vi "Test.vi"(10 "Test Controls":T1 {"Belts" scale=-1.0..1.0; "Arm" scale=-1.0..1.0; "Drive Train" scale=-1.0..1.0}, 11 "Call Context":T9) -> (0 "Loop 2 Data":T5, 1 "SubState 2":T4, 2 "Loop 1 Data":T6, 3 "SubState 1":T4, 4 "SubState 3":T4, 5 "Loop 0 Data":T7, 6 "Loop 3 Data":T3, 7 "SubState 0":T4=enum."driver control", 8 "SubState 4":T8, 9 "Test Data":T2)   [LabVIEW 2013]
uses:
  typedefs/subStates.ctl
  <vilib>/Rock Robotics/WPI/DriverStation/WPI_DriverStationDerivedRobotMode.ctl
  typedefs/singleUseSubstate.ctl
  typedefs/Loop Datatypes/Loop 0 Datatype.ctl
  typedefs/Loop Datatypes/Loop 1 Datatype.ctl
  typedefs/Loop Datatypes/Loop 2 Datatype.ctl
  typedefs/Loop Datatypes/Loop 3 Datatype.ctl
  typedefs/test/test data.ctl
  typedefs/test/test controls.ctl
  typedefs/fg_typedef.ctl
  typedefs/DevRef Type.ctl
  <vilib>/Rock Robotics/WPI/Solenoid/WPI_SolenoidGetEnum.vi
  <vilib>/Rock Robotics/WPI/Joystick/WPI_JoystickGetSetRefNum.vi
panel:
  out "JS Axis-X":dbl
  out "JS Axis-Y":dbl
  out "Exit Value":i32=-1
  # "Loop Data and Substates"
  # "Drive Loop"
  # "State Machine Master Loop"
  # "Pickup/Passing Belts Loop"
  # "Pickup/Passing Arm Loop"
  # "Pneumatics Loop"
  # "Test Code (Only Run in Test Mode)"
  # "Pneumatics"
  # "Home Encoders"
  # "Manual Override"
  # "Joystick Control"
  # "Arm Safeties"
  # "Sensors"
  # "Drive Encoders"
  # "Pneumatics Commands"
  # "Arm Encoder"
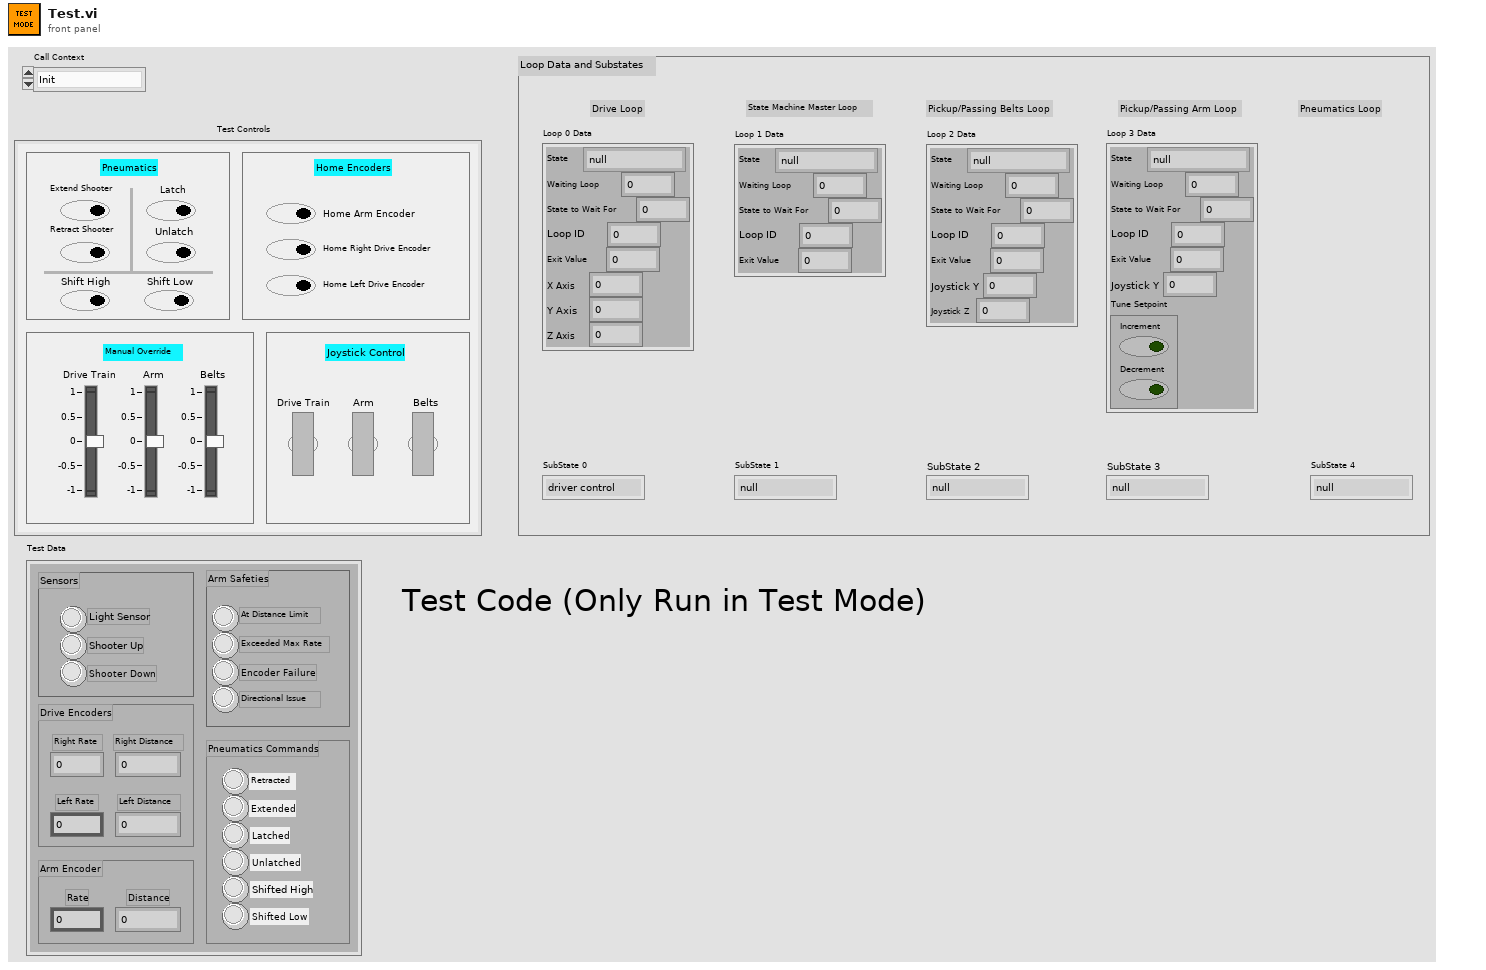
[diagram p1: front panel]
types:
  T1 = typedef "test controls.ctl" = cluster{"Drive Train":dbl, "Arm":dbl, "Belts":dbl, "Drive Train":bool, "Arm":bool, "Belts":bool, "Home Arm Encoder":bool, "Home Right Drive Encoder":bool, "Home Left Drive Encoder":bool, "Extend Shooter":bool, "Retract Shooter":bool, "Latch":bool, "Unlatch":bool, "Shift High":bool, "Shift Low":bool}
  T2 = typedef "test data.ctl" = cluster{"Light Sensor":bool, "Shooter Up":bool, "Shooter Down":bool, "Left Rate":dbl, "Left Distance":dbl, "Right Rate":dbl, "Right Distance":dbl, "Rate":dbl, "Distance":dbl, "At Distance Limit":bool, "Exceeded Max Rate":bool, "Encoder Failure":bool, "Directional Issue":bool, "Latched":bool, "Unlatched":bool, "Shifted High":bool, "Shifted Low":bool, "Extended":bool, "Retracted":bool}
  T3 = typedef "Loop 3 Datatype.ctl" = cluster{"State":T4, "Waiting Loop":i32, "State to Wait For":i32, "Loop ID":i32, "Exit Value":i32, "Joystick Y":dbl, "Tune Setpoint":cluster{"Increment":bool, "Decrement":bool}}
  T4 = typedef "subStates.ctl" = enum16{"null", "wait", "driver control", "auto", "manual override", "hold position", "rotate", "pickup", "pass", "load", "goto shoot", "shoot high goal", "shoot low goal", "cancel arm", "cancel shooter", "end", "test"}
  T5 = typedef "Loop 2 Datatype.ctl" = cluster{"State":T4, "Waiting Loop":i32, "State to Wait For":i32, "Loop ID":i32, "Exit Value":i32, "Joystick Y":dbl, "Joystick Z":dbl}
  T6 = typedef "Loop 1 Datatype.ctl" = cluster{"State":T4, "Waiting Loop":i32, "State to Wait For":i32, "Loop ID":i32, "Exit Value":i32}
  T7 = typedef "Loop 0 Datatype.ctl" = cluster{"State":T4, "Waiting Loop":i32, "State to Wait For":i32, "Loop ID":i32, "Exit Value":i32, "X Axis":dbl, "Y Axis":dbl, "Z Axis":dbl}
  T8 = typedef "singleUseSubstate.ctl" = enum16{"null", "wait", "shift high", "shift low", "extend shooter", "retract shooter", "latch", "unlatch", "end"}
  T9 = typedef "WPI_DriverStationDerivedRobotMode.ctl" = enum16{"Init", "Execute", "Stop"}
  T10 = typedef "DevRef Type.ctl" = enum16{"Shooter Solenoid", "Latch Solenoid", "Right Up Sensor", "Right Down Sensor", "Hold Sensor", "2 Ball Switch", "Arm Encoder"}
  T11 = typedef "fg_typedef.ctl" = enum16{"Get", "Set"}
  T12 = typedef "WPI_EncoderDevRef.ctl" = cluster{"DevStatus":errorcluster, "EncoderIndex":T13, "CounterIndex":T14, "DistancePerCount":dbl, "Decoding Type":T15}
  T13 = typedef "FPGA_EncoderIdx.ctl" = enum8{"Enc 0", "Enc 1", "Enc 2", "Enc 3", "Invalid"}
  T14 = typedef "FPGA_CounterCtrSystemIndex.ctl" = enum8{"Ctr 0", "Ctr 1", "Ctr 2", "Ctr 3", "Ctr 4", "Ctr 5", "Ctr 6", "Ctr 7", "Invalid"}
  T15 = typedef "WPI_EncoderType.ctl" = enum16{"1x", "2x", "4x"}
  T16 = typedef "dashboard safety status data.ctl" = cluster{"At Distance Limit":bool, "Encoder Error":bool, "Excedded Rate Limit":bool, "Encoder Directional Issue":bool}
  T17 = typedef "WPI_SolenoidDevRef.ctl" = cluster{"DevStatus":errorcluster, "Solenoid Module":T18, "Forward Solenoid Channel":T19, "Reverse Solenoid Channel":T19}
  T18 = typedef "FPGA_TypedefSolenoidModule.ctl" = enum16{"Solenoid Module 1", "Solenoid Module 2"}
  T19 = typedef "WPI_SolenoidChannel.ctl" = enum8{"Solenoid 1", "Solenoid 2", "Solenoid 3", "Solenoid 4", "Solenoid 5", "Solenoid 6", "Solenoid 7", "Solenoid 8", "Invalid"}
  T20 = typedef "WPI_DigitalInputDevRef.ctl" = cluster{"DevStatus":errorcluster, "DIO Channel":T21, "Digital Module":T22}
  T21 = typedef "FPGA_DIOChannel.ctl" = enum8{"DIO 1", "DIO 2", "DIO 3", "DIO 4", "DIO 5", "DIO 6", "DIO 7", "DIO 8", "DIO 9", "DIO 10", "DIO 11", "DIO 12", "DIO 13", "DIO 14", "Invalid"}
  T22 = typedef "FPGA_TypedefDigitalModule.ctl" = enum16{"Digital Module 1", "Digital Module 2"}
  T23 = typedef "WPI_JoystickDevRef.ctl" = cluster{"Device":T24}
  T24 = typedef "WPI_JoystickDeviceEnum.ctl" = enum16{"USB 1", "USB 2", "USB 3", "USB 4", "Kinect 1", "Kinect 2"}
  T25 = cluster{"axis 1 (x)":dbl, "axis 2 (y)":dbl, "axis 3 (throttle)":dbl, "axis 4":dbl, "axis 5":dbl, "axis 6":dbl}
  T26 = typedef "WPI_SolenoidValue.ctl" = enum16{"Off", "On", "Forward", "Reverse"}
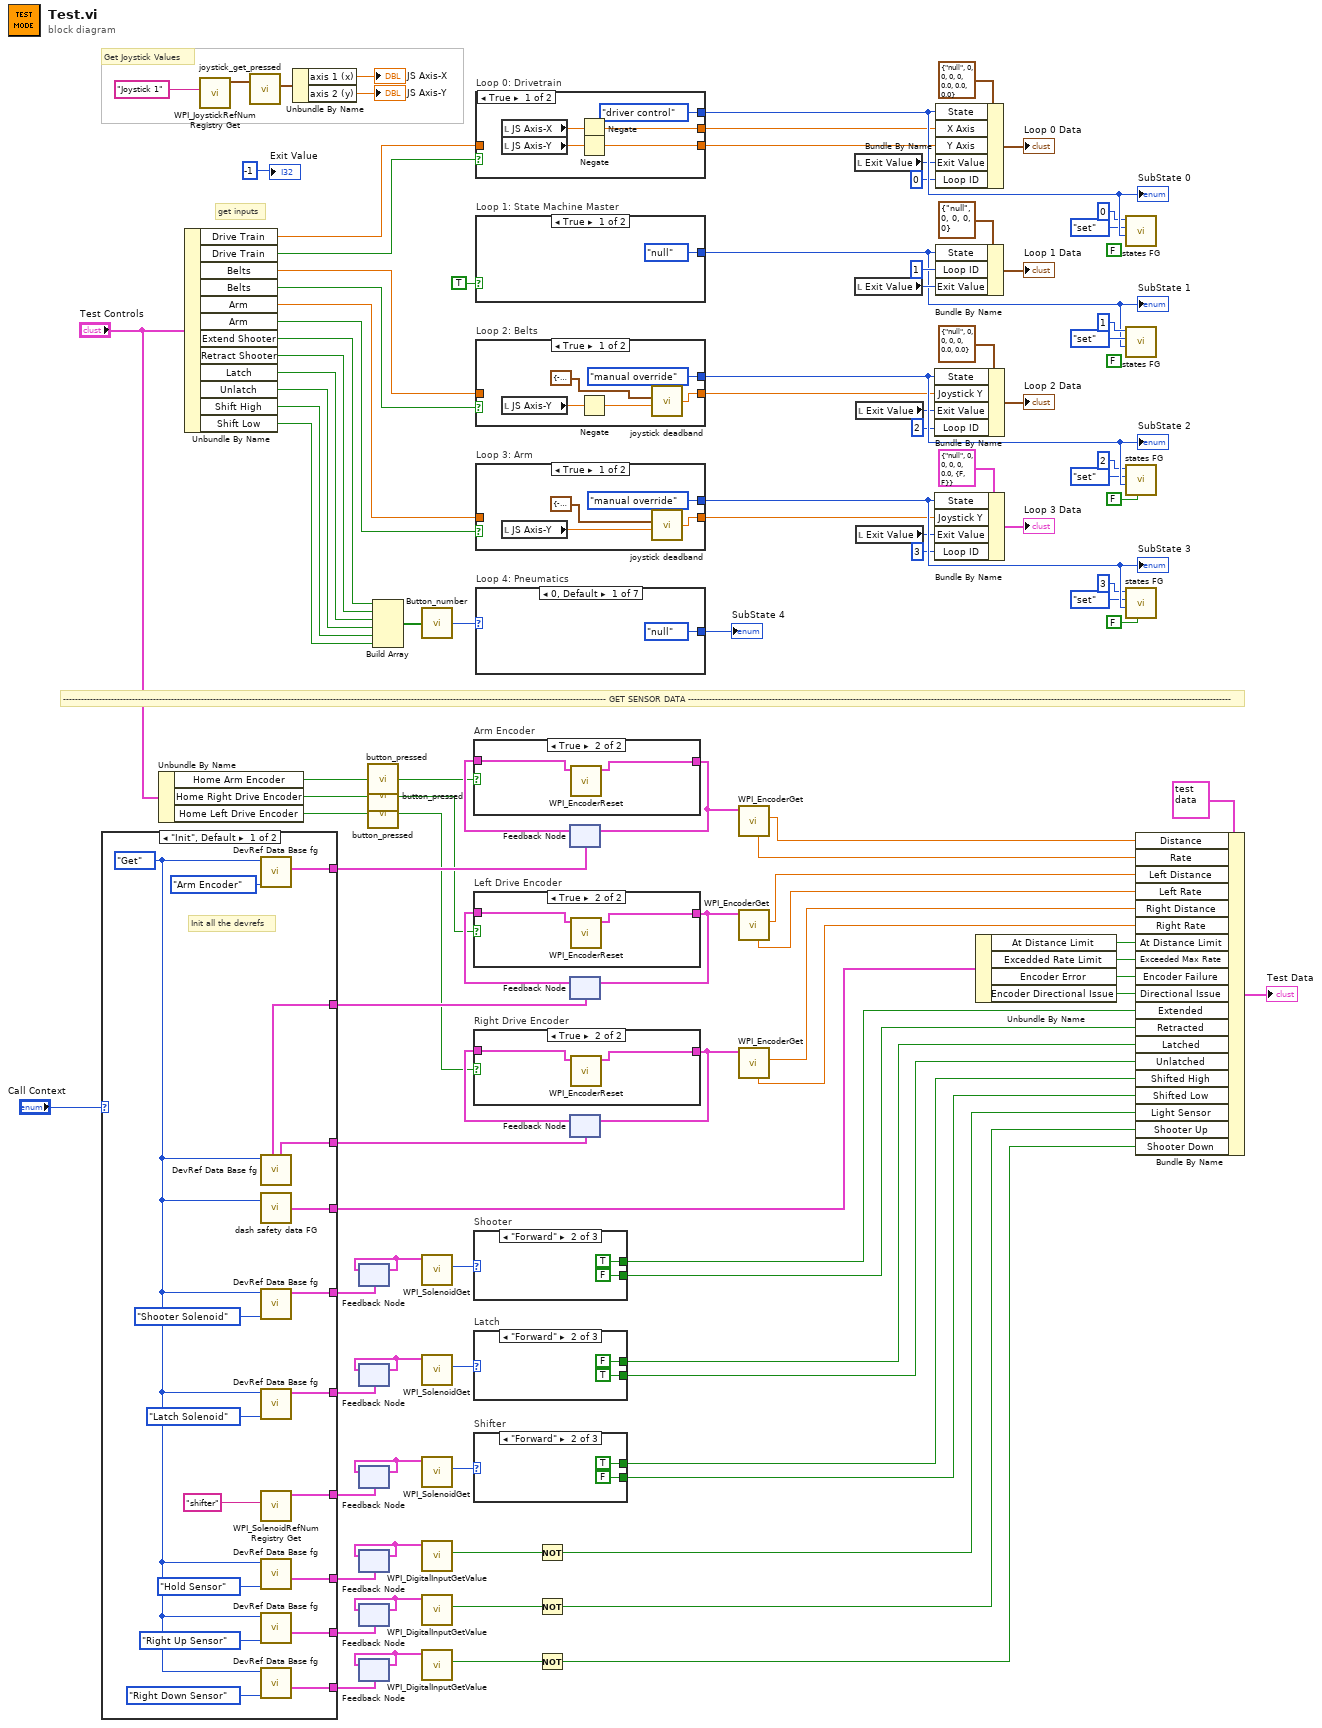
[diagram p0: block diagram]
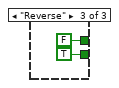
[diagram p3: hidden frame]
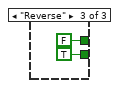
[diagram p5: hidden frame]
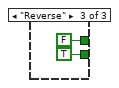
[diagram p7: hidden frame]
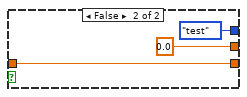
[diagram p12: hidden frame]
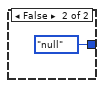
[diagram p13: hidden frame]
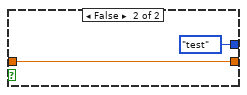
[diagram p14: hidden frame]
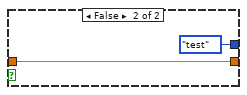
[diagram p15: hidden frame]
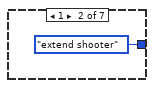
[diagram p16: hidden frame]
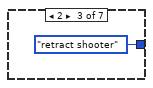
[diagram p17: hidden frame]
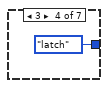
[diagram p18: hidden frame]
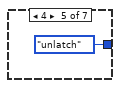
[diagram p19: hidden frame]
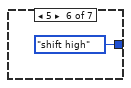
[diagram p20: hidden frame]
diagram:
  (unwired) FALSE ("exit in")
  (unwired) FALSE ("exit in")
  # "------------------------------------------------------------------------------------------------------------------------------------------------------------------------------------- GET SENSOR DATA -------------------------------------------------------------------------------------------------------------------------------------------------------------------------------------"
  # "get inputs"
  # "Get Joystick Values"
  n1 = case shown="\"Init\", Default" "Call Context" {
    tunnel: [w130 _] -> w56
    tunnel: [w129 _] -> w52
    tunnel: [w128 _] -> w51
    tunnel: [w126 _] -> w33
    tunnel: [w125 _] -> w28
    tunnel: [w124 _] -> w20
    tunnel: [w121 _] -> w17
    tunnel: [w119 _] -> w12
    tunnel: [w118 _] -> w7
    tunnel: [w115 _] -> w3
    frame "Init", Default {
      w114 = fg_typedef."Get" ("Menu")
      # "Init all the devrefs"
      n2 = call "DevRef Data Base fg.vi"("DevRef to Get"=DevRef_Type."Arm Encoder", "Menu"=w114) -> ("Selected Encoder"=w130:T12)  [unwired: 2 in, 5 out]
      n3 = call "DevRef Data Base fg.vi"("Menu"=w114) -> ("right drive encoder"=w128:T12, "left drive encoder"=w129:T12)  [unwired: 3 in, 4 out]
      n4 = call "dash safety data FG.vi"("Menu"=w114) -> ("Safety Data Out"=w126:T16)  [unwired: 1 in]
      n5 = call "DevRef Data Base fg.vi"("DevRef to Get"=DevRef_Type."Shooter Solenoid", "Menu"=w114) -> ("Selected Solenoid"=w125:T17)  [unwired: 2 in, 5 out]
      n6 = call "DevRef Data Base fg.vi"("DevRef to Get"=DevRef_Type."Latch Solenoid", "Menu"=w114) -> ("Selected Solenoid"=w124:T17)  [unwired: 2 in, 5 out]
      n7 = call <vilib>:"WPI_SolenoidRefNum Registry Get.vi"("refnum name"="shifter") -> ("SolenoidDevRef"=w121:T17)  [unwired: 9 in, 1 out]
      n8 = call "DevRef Data Base fg.vi"("DevRef to Get"=DevRef_Type."Hold Sensor", "Menu"=w114) -> ("Selected Sensor"=w119:T20)  [unwired: 2 in, 5 out]
      n9 = call "DevRef Data Base fg.vi"("DevRef to Get"=DevRef_Type."Right Up Sensor", "Menu"=w114) -> ("Selected Sensor"=w118:T20)  [unwired: 2 in, 5 out]
      n10 = call "DevRef Data Base fg.vi"("DevRef to Get"=DevRef_Type."Right Down Sensor", "Menu"=w114) -> ("Selected Sensor"=w115:T20)  [unwired: 2 in, 5 out]
    }
    frame "Execute", "Stop" {
      # "do nothing"
    }
  }
  n11 = Unbundle By Name("Test Controls") -> ("Home Arm Encoder"=w50:bool, "Home Right Drive Encoder"=w48:bool, "Home Left Drive Encoder"=w46:bool)
  n12 = Unbundle By Name("Test Controls") -> ("Drive Train"=w72:dbl, "Drive Train"=w73:bool, "Belts"=w85:dbl, "Belts"=w86:bool, "Arm"=w104:dbl, "Arm"=w105:bool, "Extend Shooter"=w63:bool, "Retract Shooter"=w62:bool, "Latch"=w61:bool, "Unlatch"=w60:bool, "Shift High"=w59:bool, "Shift Low"=w58:bool)
  n13 = call <vilib>:"WPI_JoystickRefNum Registry Get.vi"("refnum name"="Joystick 1") -> ("JoystickDevRef"=w100:T23)  [unwired: 9 in, 1 out]
  n14 = call "joystick_get_pressed.vi"("JoystickDevRef 2"=w100) -> ("Axes"=w98:T25)  [unwired: 1 in, 3 out]
  n15 = Unbundle By Name(w98) -> ("axis 1 (x)"=→"JS Axis-X":dbl, "axis 2 (y)"=→"JS Axis-Y":dbl)
  n16 = feedback #1(w28) -> (w26:T17)
  n17 = feedback-in #1(w26) -> ()
  n18 = feedback #2(w20) -> (w21:T17)
  n19 = feedback-in #2(w21) -> ()
  n20 = feedback #3(w17) -> (w16:T17)
  n21 = feedback-in #3(w16) -> ()
  n22 = feedback #4(w12) -> (w11:T20)
  n23 = feedback-in #4(w11) -> ()
  n24 = feedback #5(w7) -> (w8:T20)
  n25 = feedback-in #5(w8) -> ()
  n26 = feedback #6(w3) -> (w2:T20)
  n27 = feedback-in #6(w2) -> ()
  n28 = call "button_pressed.vi"("Button In"=w50) -> ("Button Pressed?"=w49:bool)
  n29 = call "button_pressed.vi"("Button In"=w48) -> ("Button Pressed?"=w47:bool)
  n30 = call "button_pressed.vi"("Button In"=w46) -> ("Button Pressed?"=w45:bool)
  n31 = Build Array(w63, w62, w61, w60, w59, w58) -> (w110:bool[])
  n32 = call "Button_number.vi"("Button Array"=w110) -> ("Button Pressed"=w109:i32)
  n33 = call-poly <vilib>:"WPI_SolenoidGet.vi"("SolenoidDevRef"=w26) -> ("Value"=w25:T26)  [unwired: 8 in, 2 out]
  n34 = call-poly <vilib>:"WPI_SolenoidGet.vi"("SolenoidDevRef"=w21) -> ("Value"=w22:T26)  [unwired: 8 in, 2 out]
  n35 = call-poly <vilib>:"WPI_SolenoidGet.vi"("SolenoidDevRef"=w16) -> ("Value"=w15:T26)  [unwired: 8 in, 2 out]
  n36 = call <vilib>:"WPI_DigitalInputGetValue.vi"("DigitalInputDevRef"=w11) -> ("Value"=w10:bool)  [unwired: 8 in, 2 out]
  n37 = call <vilib>:"WPI_DigitalInputGetValue.vi"("DigitalInputDevRef"=w8) -> ("Value"=w6:bool)  [unwired: 8 in, 2 out]
  n38 = call <vilib>:"WPI_DigitalInputGetValue.vi"("DigitalInputDevRef"=w2) -> ("Value"=w4:bool)  [unwired: 8 in, 2 out]
  n39 = case "Shooter" shown="\"Forward\"" w25 {
    tunnel: [_ TRUE FALSE] -> w24
    tunnel: [_ FALSE TRUE] -> w23
    frame "Off", Default {
    }
    frame "Forward" {
    }
    frame "Reverse" {
    }
  }
  n40 = case "Latch" shown="\"Forward\"" w22 {
    tunnel: [_ FALSE FALSE] -> w19
    tunnel: [_ TRUE TRUE] -> w18
    frame "Off", Default {
    }
    frame "Forward" {
    }
    frame "Reverse" {
    }
  }
  n41 = case "Shifter" shown="\"Forward\"" w15 {
    tunnel: [_ TRUE FALSE] -> w14
    tunnel: [_ FALSE TRUE] -> w13
    frame "Off", Default {
    }
    frame "Forward" {
    }
    frame "Reverse" {
    }
  }
  n42 = case "Loop 0: Drivetrain" shown="True" w73 {
    tunnel: w72 -> [_ w150]
    tunnel: [w144 w150] -> w64
    tunnel: [subStates."driver control" ("State") subStates."test" ("State")] -> w113
    tunnel: [w145 0.0 ("JS Axis-X")] -> w65
    frame True {
      n43 = local read "JS Axis-X"() -> (w147:dbl)
      n44 = local read "JS Axis-Y"() -> (w146:dbl)
      n45 = Negate(x=w147) -> (-x=w145:dbl)
      n46 = Negate(x=w146) -> (-x=w144:dbl)
    }
    frame False {
    }
  }
  "SubState 0" <- w113
  n47 = case "Loop 1: State Machine Master" shown="True" TRUE {
    tunnel: [subStates."null" ("State") subStates."null" ("State")] -> w74
    frame True {
    }
    frame False {
    }
  }
  "SubState 1" <- w74
  n48 = case "Loop 2: Belts" shown="True" w86 {
    tunnel: w85 -> [_ w159]
    tunnel: [w157 w159] -> w88
    tunnel: [subStates."manual override" ("State") subStates."test" ("State")] -> w112
    frame True {
      n49 = local read "JS Axis-Y"() -> (w156:dbl)
      n50 = Negate(x=w156) -> (-x=w154:dbl)
      n51 = call "joystick deadband.vi"("Joystick In"=w154, "Deadband Range"=cluster{"Deadband Min":dbl, "Deadband Max":dbl} {"Deadband Min"=-0.09, "Deadband Max"=0.09}) -> ("Joystick Out"=w157:dbl)  [unwired: 4 in]
    }
    frame False {
    }
  }
  "SubState 2" <- w112
  n52 = case "Loop 3: Arm" shown="True" w105 {
    tunnel: w104 -> [_ w166]
    tunnel: [w163 w166] -> w102
    tunnel: [subStates."manual override" ("State") subStates."test" ("State")] -> w111
    frame True {
      n53 = local read "JS Axis-Y"() -> (w162:dbl)
      n54 = call "joystick deadband.vi"("Joystick In"=w162, "Deadband Range"=cluster{"Deadband Min":dbl, "Deadband Max":dbl} {"Deadband Min"=-0.09, "Deadband Max"=0.09}) -> ("Joystick Out"=w163:dbl)  [unwired: 4 in]
    }
    frame False {
    }
  }
  "SubState 3" <- w111
  n55 = case "Loop 4: Pneumatics" shown="0, Default" w109 {
    tunnel: [singleUseSubstate."null" ("SubState 4") singleUseSubstate."extend shooter" ("SubState 4") singleUseSubstate."retract shooter" ("SubState 4") singleUseSubstate."latch" ("SubState 4") singleUseSubstate."unlatch" ("SubState 4") singleUseSubstate."shift high" ("SubState 4") singleUseSubstate."shift low" ("SubState 4")] -> w108
    frame 0, Default {
    }
    frame 1 {
    }
    frame 2 {
    }
    frame 3 {
    }
    frame 4 {
    }
    frame 5 {
    }
    frame 6 {
    }
  }
  "SubState 4" <- w108
  n56 = Not(x=w10) -> (.not. x?=w9:bool)
  n57 = Not(x=w6) -> (.not. x?=w5:bool)
  n58 = Not(x=w4) -> (.not. x?=w1:bool)
  n59 = feedback #7(w56) -> (w55:T12)
  n60 = case "Arm Encoder" shown="True" w49 {
    tunnel: w55 -> [w174 w176]
    tunnel: [w174 w175] -> w42
    frame False {
    }
    frame True {
      n61 = call <vilib>:"WPI_EncoderReset.vi"("EncoderDevRef"=w176) -> ("EncoderDevRef"=w175:T12)  [unwired: 9 in, 1 out]
    }
  }
  n62 = feedback-in #7(w42) -> ()
  n63 = feedback #8(w52) -> (w54:T12)
  n64 = case "Left Drive Encoder" shown="True" w47 {
    tunnel: w54 -> [w177 w179]
    tunnel: [w177 w178] -> w41
    frame False {
    }
    frame True {
      n65 = call <vilib>:"WPI_EncoderReset.vi"("EncoderDevRef"=w179) -> ("EncoderDevRef"=w178:T12)  [unwired: 9 in, 1 out]
    }
  }
  n66 = feedback-in #8(w41) -> ()
  n67 = feedback #9(w51) -> (w53:T12)
  n68 = case "Right Drive Encoder" shown="True" w45 {
    tunnel: w53 -> [w180 w182]
    tunnel: [w180 w181] -> w40
    frame False {
    }
    frame True {
      n69 = call <vilib>:"WPI_EncoderReset.vi"("EncoderDevRef"=w182) -> ("EncoderDevRef"=w181:T12)  [unwired: 9 in, 1 out]
    }
  }
  n70 = feedback-in #9(w40) -> ()
  n71 = call <vilib>:"WPI_EncoderGet.vi"("EncoderDevRef"=w42) -> ("Distance"=w39:dbl, "Rate"=w38:dbl)  [unwired: 5 in, 4 out]
  n72 = call <vilib>:"WPI_EncoderGet.vi"("EncoderDevRef"=w41) -> ("Distance"=w37:dbl, "Rate"=w36:dbl)  [unwired: 5 in, 4 out]
  n73 = call <vilib>:"WPI_EncoderGet.vi"("EncoderDevRef"=w40) -> ("Distance"=w35:dbl, "Rate"=w34:dbl)  [unwired: 5 in, 4 out]
  n74 = local read "Exit Value"() -> (w69:i32)
  n75 = local read "Exit Value"() -> (w82:i32)
  n76 = local read "Exit Value"() -> (w89:i32)
  n77 = local read "Exit Value"() -> (w99:i32)
  n78 = Bundle By Name(cluster=T5 {"State"=enum."null", "Waiting Loop"=0, "State to Wait For"=0, "Loop ID"=0, "Exit Value"=0, "Joystick Y"=0.0, "Joystick Z"=0.0} ("Loop 2 Data"), "State"=w112, "Joystick Y"=w88, "Exit Value"=w89, "Loop ID"=2) -> (→"Loop 2 Data":T5)
  n79 = Bundle By Name(cluster=T3 {"State"=enum."null", "Waiting Loop"=0, "State to Wait For"=0, "Loop ID"=0, "Exit Value"=0, "Joystick Y"=0.0, "Tune Setpoint"={"Increment"=FALSE, "Decrement"=FALSE}} ("Loop 3 Data"), "State"=w111, "Joystick Y"=w102, "Exit Value"=w99, "Loop ID"=3) -> (→"Loop 3 Data":T3)
  n80 = Bundle By Name(cluster=T7 {"State"=enum."null", "Waiting Loop"=0, "State to Wait For"=0, "Loop ID"=0, "Exit Value"=0, "X Axis"=0.0, "Y Axis"=0.0, "Z Axis"=0.0} ("Loop 0 Data"), "State"=w113, "X Axis"=w65, "Y Axis"=w64, "Exit Value"=w69, "Loop ID"=0) -> (→"Loop 0 Data":T7)
  n81 = Bundle By Name(cluster=T6 {"State"=enum."null", "Waiting Loop"=0, "State to Wait For"=0, "Loop ID"=0, "Exit Value"=0} ("Loop 1 Data"), "State"=w74, "Loop ID"=1, "Exit Value"=w82) -> (→"Loop 1 Data":T6)
  n82 = Unbundle By Name(w33) -> ("At Distance Limit"=w32:bool, "Excedded Rate Limit"=w31:bool, "Encoder Error"=w30:bool, "Encoder Directional Issue"=w29:bool)
  n83 = call "states FG.vi"("subState in"=w113, "menu (get)"=enum16{"set", "get"}."set", "Loop ID"=0) -> ()  [unwired: 5 in, 4 out]
  n84 = call "states FG.vi"("subState in"=w74, "menu (get)"=enum16{"set", "get"}."set", "Loop ID"=1) -> ()  [unwired: 5 in, 4 out]
  n85 = call "states FG.vi"("exit in"=FALSE, "subState in"=w112, "menu (get)"=enum16{"set", "get"}."set", "Loop ID"=2) -> ()  [unwired: 4 in, 4 out]
  n86 = call "states FG.vi"("exit in"=FALSE, "subState in"=w111, "menu (get)"=enum16{"set", "get"}."set", "Loop ID"=3) -> ()  [unwired: 4 in, 4 out]
  n87 = Bundle By Name(cluster=T2 {"Light Sensor"=FALSE, "Shooter Up"=FALSE, "Shooter Down"=FALSE, "Left Rate"=0.0, "Left Distance"=0.0, "Right Rate"=0.0, "Right Distance"=0.0, "Rate"=0.0, "Distance"=0.0, "At Distance Limit"=FALSE, "Exceeded Max Rate"=FALSE, "Encoder Failure"=FALSE, "Directional Issue"=FALSE, "Latched"=FALSE, "Unlatched"=FALSE, "Shifted High"=FALSE, "Shifted Low"=FALSE, "Extended"=FALSE, "Retracted"=FALSE} ("Test Data"), "Distance"=w39, "Rate"=w38, "Left Distance"=w37, "Left Rate"=w36, "Right Distance"=w35, "Right Rate"=w34, "At Distance Limit"=w32, "Exceeded Max Rate"=w31, "Encoder Failure"=w30, "Directional Issue"=w29, "Extended"=w24, "Retracted"=w23, "Latched"=w19, "Unlatched"=w18, "Shifted High"=w14, "Shifted Low"=w13, "Light Sensor"=w9, "Shooter Up"=w5, "Shooter Down"=w1) -> (→"Test Data":T2)
  "Exit Value" <- -1 ("Exit Value")
